vi "AMPL_OFFSET(SA).vi"(4 "Timeout":u32=3000, 6 "RO(T)":bool, 7 "RlevOffset":dbl format="%#_13g", 8 "error in":errorcluster {"code" format="%.0x"}, 11 "Session In":refnum<visa-resource-name>="GPIB0::16::INSTR") -> (0 "error out":errorcluster {"code" format="%.0x"}, 2 "OFFSET":dbl, 3 "Session Out":refnum<visa-resource-name>)   [LabVIEW 2018]
doc: "Launches the Instrument I/O Assistant, which you can use to communicate with message-based instruments and graphically parse the response. For example you can communicate with an instrument that uses a serial, Ethernet, or GPIB interface."
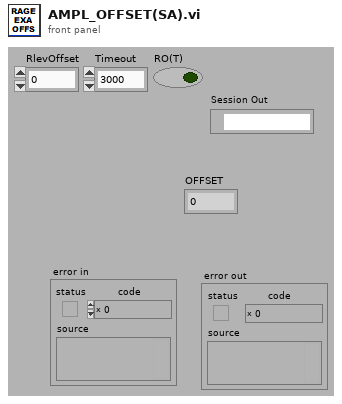
[diagram p1: front panel]
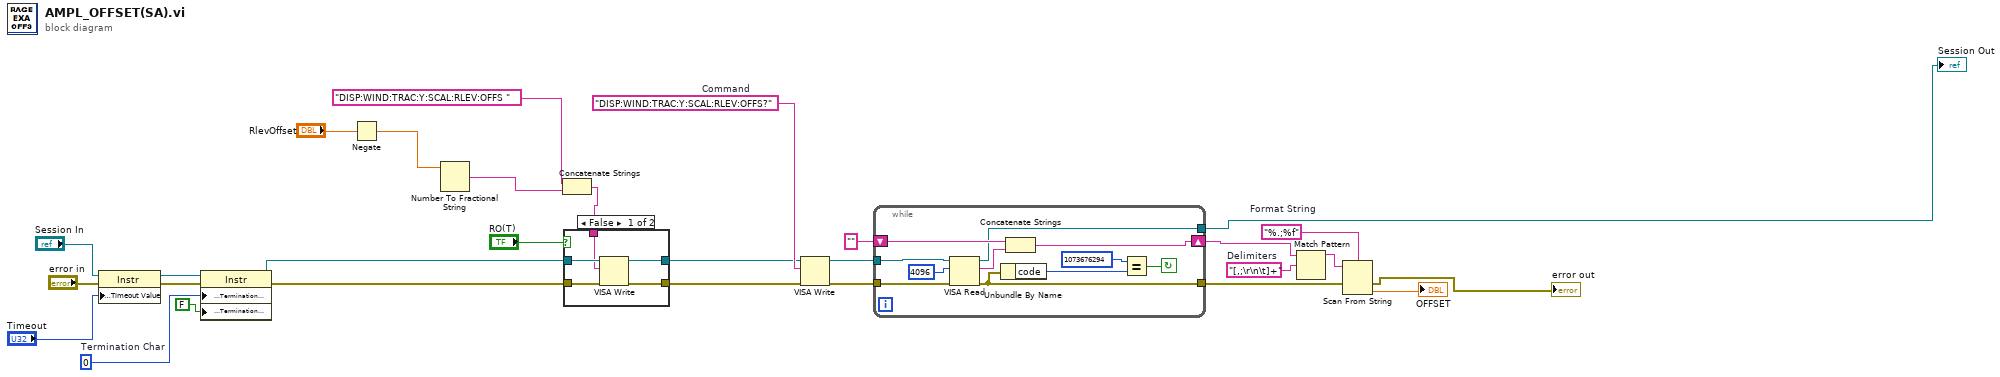
[diagram p0: block diagram]
diagram:
  w15 = "[,;\r\n\t]+"  # Delimiters
  w16 = "%.;%f"  # Format String
  w19 = "DISP:WIND:TRAC:Y:SCAL:RLEV:OFFS?"  # Command
  w26 = u8 0  # Termination Char
  n1 = property class="Instr"(reference="Session In", error in="error in", "General Settings:Timeout Value"="Timeout") -> (reference out=w25:refnum<visa-resource-name>, error out=w27:errorcluster)
  n2 = property class="Instr"(reference=w25, error in=w27, "Message Based Settings:Termination Character"=w26, "Message Based Settings:Termination Character Enable"=FALSE ("enable")) -> (reference out=w14:refnum<visa-resource-name>, error out=w13:errorcluster)
  n3 = Negate(x="RlevOffset") -> (-x=w1:dbl)
  n4 = Number To Fractional String(number=w1) -> (F-format string=w10:string)  [unwired: 3 in]
  n5 = Concatenate Strings("DISP:WIND:TRAC:Y:SCAL:RLEV:OFFS " ("StaticText"), w10) -> (w9:string)
  n6 = case shown="False" "RO(T)" {
    tunnel: w14 -> [w34 w36]
    tunnel: w13 -> [w33 w35]
    tunnel: w9 -> [w32 _]
    tunnel: [w31 w35] -> w4
    tunnel: [w30 w36] -> w3
    frame False {
      n7 = VISA Write(VISA resource name=w34, write buffer=w32, error in (no error)=w33) -> (VISA resource name out=w30:refnum<visa-resource-name>, error out=w31:errorcluster)  [unwired: 1 out]
    }
    frame True {
    }
  }
  n8 = VISA Write(VISA resource name=w3, write buffer=w19, error in (no error)=w4) -> (VISA resource name out=w23:refnum<visa-resource-name>, error out=w22:errorcluster)  [unwired: 1 out]
  n9 = while {
    tunnel: w23 -> [w44]
    shift-right: [w38] -> w18
    shift-left: "" -> [w43]
    tunnel: w22 -> [w41]
    tunnel: [w40] -> w21
    tunnel: [w37] -> w6
    stop <- w39 continue-if-true
    n10 = VISA Read(VISA resource name=w44, byte count=u32 4096 ("byte count (0)"), error in (no error)=w41) -> (VISA resource name out=w37:refnum<visa-resource-name>, read buffer=w42:string, error out=w40:errorcluster)  [unwired: 1 out]
    n11 = Unbundle By Name(w40) -> ("code"=w46:i32)
    n12 = Concatenate Strings(w43, w42) -> (w38:string)
    n13 = Equal?(x=1073676294, y=w46) -> (x = y?=w39:bool)
  }
  "Session Out" <- w6
  n14 = Match Pattern(string=w18, regular expression=w15) -> (before substring=w17:string)  [unwired: 1 in, 3 out]
  n15 = Scan From String(format string=w16, input string=w17, error in=w21) -> (error out=→"error out":errorcluster, output 1=→"OFFSET":dbl)  [unwired: 2 in, 2 out]
